vi "Precision.vi"(8 "Precise?":bool, 9 "Percent Power":dbl, 10 "Number In":dbl) -> (2 "Number Out":dbl)   [LabVIEW 2015]
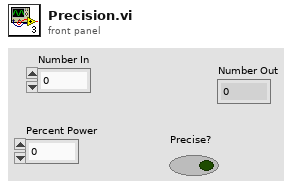
[diagram p1: front panel]
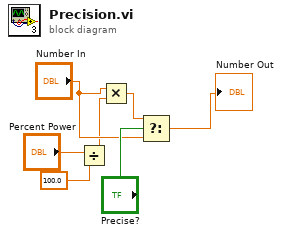
[diagram p0: block diagram]
diagram:
  n1 = Divide(x="Percent Power", y=100.0) -> (x/y=w4:dbl)
  n2 = Multiply(x="Number In", y=w4) -> (x*y=w1:dbl)
  n3 = Select(t=w1, s="Precise?", f="Number In") -> (s? t:f=→"Number Out":dbl)
